vi "CleanUp Word Report.vi"(6 "close report? (T)":bool=TRUE, 8 "error in (no error)":errorcluster, 11 "Word_Report in":refnum<class "Word_Report.lvclass">) -> (0 "error out":errorcluster, 3 "Word_Report out":refnum<class "Word_Report.lvclass">)   [LabVIEW 2018, in "WordReportGeneration.lvlib" / "Word_Report.lvclass"]
uses:
  Word_Report.lvclass
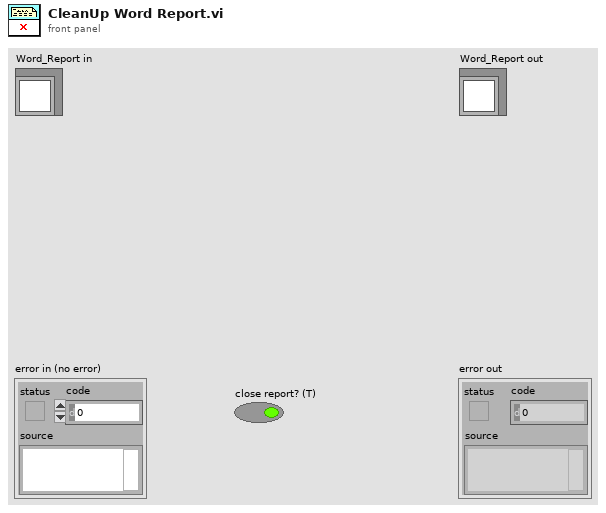
[diagram p1: front panel]
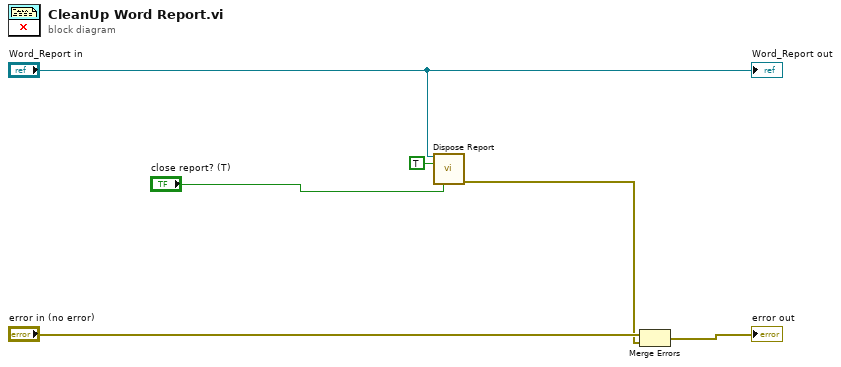
[diagram p0: block diagram]
diagram:
  n1 = call-dynamic "Dispose Report.vi"("report in"="Word_Report in", "wait until printing completed? (T)"=TRUE, "close report? (T)"="close report? (T)") -> ("error out"=w2:errorcluster)  [unwired: 12 in]
  n2 = Merge Errors("error in (no error)", w2) -> (→"error out":errorcluster)
  "Word_Report out" <- "Word_Report in"
